vi "子VI-深度学习自动检测结果分析.vi"(2 "临界Z值":i32, 4 "临界面积百分比值":dbl, 6 "预测图片保存路径":path, 12 "产品规格":cluster{"产品长度（周长）（mm）":dbl, "产品宽度（母线长）（mm）":dbl}) -> (14 "弥散类检测结果":string[][](table), 17 "Threshold Image":T2(plugin-control), 18 "misan":T2(plugin-control), 19 "分层类检测结果":string[][](table))   [LabVIEW 2018]
uses:
  <vilib>/vision/NI_Vision_Development_Module.lvlib
panel:
  in  "Tab Control":T1
  out "?":T2(plugin-control)
  in  "格式字符串 3":string="%f"
  in  "分隔符（'\\'代码显示） 2":string="\t"
  out "弥散和分层临界灰度值":i64
  out "弥散缺陷个数":i32
  out "分层缺陷个数":i32
  out "合格？ 弥散类":string="fencengThreshold"
  out "合格？分层类":string="fencengThreshold"
  out "弥散测量结果":dbl[][](array[numeric]) format="%.2f"
  out "面积 (pixels)":i32
  in  "格式字符串 2":string="%f"
  in  "分隔符（'\\'代码显示）":string="\t"
  out "分层测量结果":dbl[][](array[numeric]) format="%.2f"
  out "缺陷初步分类的临界值":sgl format="%#.3f"
  # "所选区域信息"
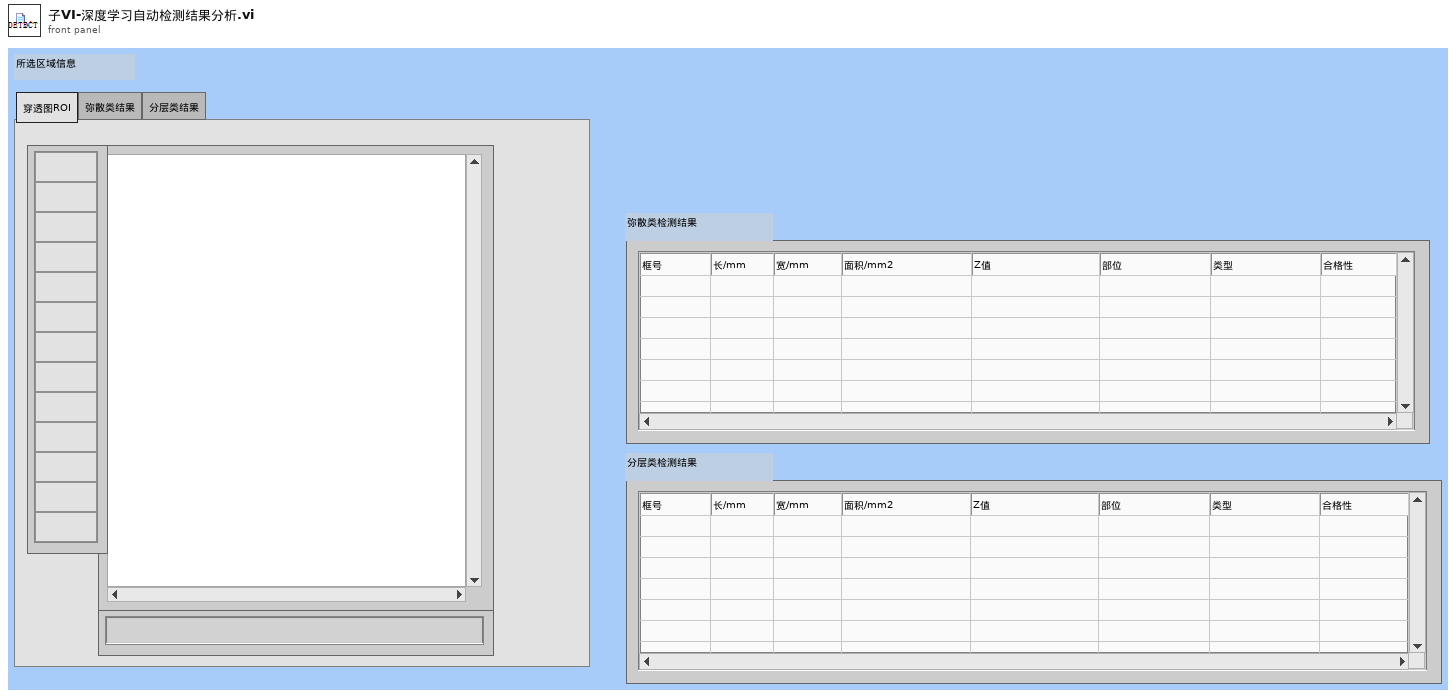
[diagram p1: front panel]
types:
  T1 = typedef "控件2.ctl" = enum32{"穿透图ROI", "弥散类结果", "分层类结果"}
  T2 = typedef "IMAQ Image.ctl" = refnum<image>
  T3 = typedef "Image Type" = u32
  T4 = typedef "Particle Parameters" = i32
  T5 = cluster{"Measurement Parameter":T4, "Range Lower Value":dbl, "Range Upper Value":dbl, "Range":bool, "Measurement Type":bool}[]
  T6 = cluster{"histogram":u32[], "Minimal Value":sgl, "Maximal Value":sgl, "Starting Value":sgl, "Interval Width":sgl, "Mean Value":sgl, "Standard  Variation":sgl, "Area (pixels)":i32}
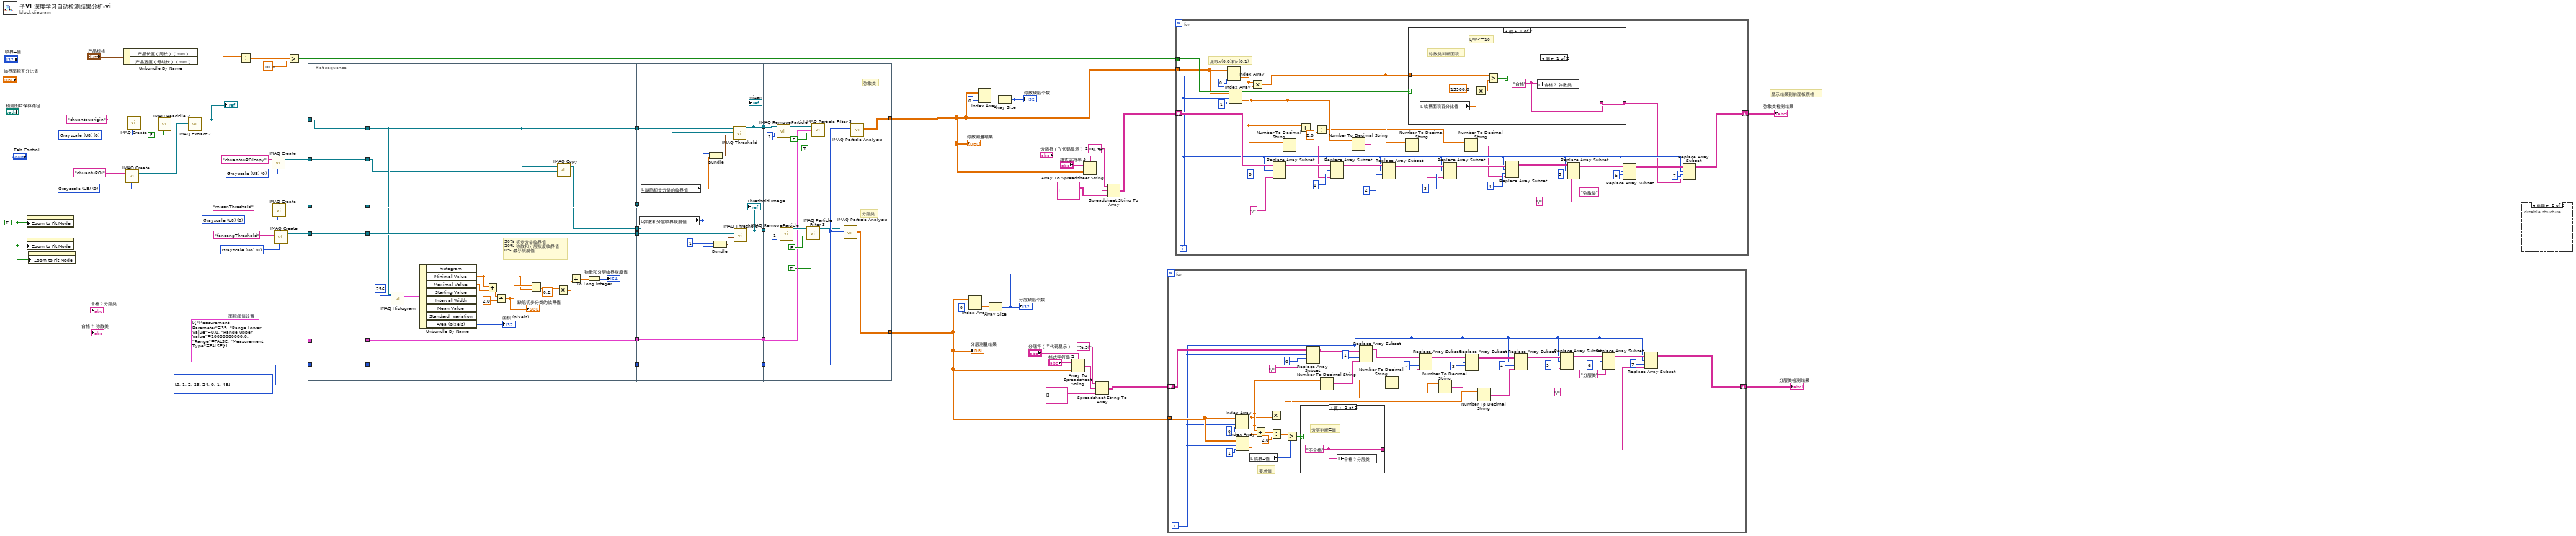
[diagram p0: block diagram]
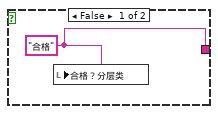
[diagram p2: hidden frame]
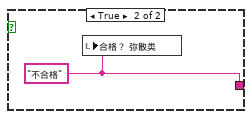
[diagram p3: hidden frame]
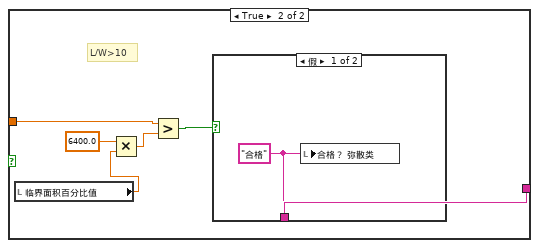
[diagram p4: hidden frame]
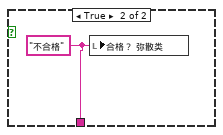
[diagram p5: hidden frame]
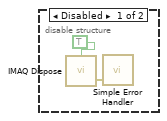
[diagram p6: hidden frame]
diagram:
  w1 = T3 0 items=["Grayscale (U8)", "Grayscale (I16)", "Grayscale (SGL)", "Complex (CSG)", "RGB (U32)", "HSL (U32)", "RGB (U64)", "Grayscale (U16)"] ("Image Type")
  w6 = TRUE ("Zoom to Fit Mode")
  w47 = T3 0 items=["Grayscale (U8)", "Grayscale (I16)", "Grayscale (SGL)", "Complex (CSG)", "RGB (U32)", "HSL (U32)", "RGB (U64)", "Grayscale (U16)"] ("Image Type")
  w48 = T3 0 items=["Grayscale (U8)", "Grayscale (I16)", "Grayscale (SGL)", "Complex (CSG)", "RGB (U32)", "HSL (U32)", "RGB (U64)", "Grayscale (U16)"] ("Image Type")
  w51 = T3 0 items=["Grayscale (U8)", "Grayscale (I16)", "Grayscale (SGL)", "Complex (CSG)", "RGB (U32)", "HSL (U32)", "RGB (U64)", "Grayscale (U16)"] ("Image Type")
  w29 = i32[] [0, 1, 2, 23, 24, 0, 1, 48] items=["Bounding Rect Width", "Bounding Rect Height"] ("Pixel Measurements")
  w33 = T5 [{"Measurement Parameter"=35, "Range Lower Value"=0.0, "Range Upper Value"=10000000000.0, "Range"=FALSE, "Measurement Type"=FALSE}]  # 面积阈值设置
  w65 = T3 0 items=["Grayscale (U8)", "Grayscale (I16)", "Grayscale (SGL)", "Complex (CSG)", "RGB (U32)", "HSL (U32)", "RGB (U64)", "Grayscale (U16)"] ("Image Type")
  # "显示结果到前面板表格"
  n1 = property class="ImageControl"("Zoom to Fit Mode"=w6) -> ()  [unwired: 2 in, 2 out]
  n2 = property class="ImageControl"("Zoom to Fit Mode"=w6) -> ()  [unwired: 2 in, 2 out]
  n3 = property class="ImageControl"("Zoom to Fit Mode"=w6) -> ()  [unwired: 2 in, 2 out]
  n4 = Unbundle By Name("产品规格") -> ("产品长度（周长）（mm）"=w59:dbl, "产品宽度（母线长）（mm）"=w58:dbl)
  n5 = call "IMAQ Create"("Image Name"="chuantuROI", "Image Type"=w51) -> ("New Image"=w50:T2)  [unwired: 3 in, 1 out]
  n6 = call "IMAQ Create"("Image Name"="chuantouorigin", "Image Type"=w65) -> ("New Image"=w53:T2)  [unwired: 3 in, 1 out]
  n7 = call "IMAQ ReadFile 2"("Use File Path Image Type"=FALSE, "File Path"="预测图片保存路径", "Image"=w53) -> ("Image Out"=w54:T2)  [unwired: 4 in, 4 out]
  n8 = call "IMAQ Extract 2"("Image Dst"=w50, "Image Src"=w54) -> ("Image Dst Out"=w9:T2)  [unwired: 8 in, 1 out]
  "?" <- w9
  n9 = Divide(x=w59, y=w58) -> (x/y=w62:dbl)
  n10 = call "IMAQ Create"("Image Name"="chuantouROIcopy", "Image Type"=w1) -> ("New Image"=w4:T2)  [unwired: 3 in, 1 out]
  n11 = call "IMAQ Create"("Image Name"="misanThreshold", "Image Type"=w47) -> ("New Image"=w40:T2)  [unwired: 3 in, 1 out]
  n12 = call "IMAQ Create"("Image Name"="fencengThreshold", "Image Type"=w48) -> ("New Image"=w38:T2)  [unwired: 3 in, 1 out]
  n13 = Greater?(x=w62, y=10.0) -> (0:w57:bool)
  n14 = flat-sequence {
    tunnel: w9 -> [w68]
    tunnel: w40 -> [w72]
    tunnel: [w72] -> w41
    tunnel: [w71] -> w39
    tunnel: w38 -> [w71]
    tunnel: [w70] -> w34
    tunnel: w33 -> [w70]
    tunnel: [w69] -> w30
    tunnel: w29 -> [w69]
    tunnel: [w68] -> w7
    tunnel: w4 -> [w67]
    tunnel: [w67] -> w3
    tunnel: [w92] -> w42
    tunnel: [w91] -> w37
    tunnel: [w86] -> w32
    tunnel: [w85] -> w28
    tunnel: w30 -> [w85]
    tunnel: w34 -> [w86]
    tunnel: w39 -> [w91]
    tunnel: w41 -> [w92]
    tunnel: [w75] -> w8
    tunnel: w7 -> [w75]
    tunnel: [w74] -> w5
    tunnel: w3 -> [w73]
    tunnel: w42 -> [w105]
    tunnel: w37 -> [w104]
    tunnel: [w94] -> w36
    tunnel: [w95] -> w35
    tunnel: w32 -> [w103]
    tunnel: [w103] -> w31
    tunnel: w28 -> [w102]
    tunnel: [w102] -> w27
    tunnel: w8 -> [w96]
    tunnel: w5 -> [w93]
    tunnel: [w108] -> w12
    tunnel: [w115] -> w20
    tunnel: w36 -> [w114]
    tunnel: w35 -> [w113]
    tunnel: w31 -> [w112]
    tunnel: w27 -> [w111]
    frame #0 {
    }
    frame #1 {
      # "50% 初步分类临界值\n20% 弥散和分层灰度临界值\n0% 最小灰度值"
      n15 = call "IMAQ Histogram"("Number of Classes"=256, "Image"=w75) -> ("Histogram Report"=w89:T6)  [unwired: 8 in, 1 out]
      n16 = Unbundle By Name(w89) -> ("Minimal Value"=w77:sgl, "Maximal Value"=w83:sgl, "Area (pixels)"=→"面积 (pixels)":i32)  [unwired: 5 out]
      n17 = Add(x=w77, y=w83) -> (x+y=w82:sgl)
      n18 = Divide(x=w82, y=sgl 2.0) -> (x/y=w81:sgl)
      "缺陷初步分类的临界值" <- w81
      n19 = Subtract(x=w81, y=w77) -> (x-y=w79:sgl)
      n20 = Multiply(x=w79, y=0.2) -> (x*y=w78:dbl)
      n21 = call "IMAQ Copy"("Image Dst"=w73, "Image Src"=w75) -> ("Image Dst Out"=w74:T2)  [unwired: 4 in, 1 out]
      n22 = Add(x=w77, y=w78) -> (x+y=w76:dbl)
      n23 = To Long Integer(number=w76) -> (32bit integer=→"弥散和分层临界灰度值":i32)
    }
    frame #2 {
      n24 = local read "弥散和分层临界灰度值"() -> (w98:i64)
      n25 = local read "缺陷初步分类的临界值"() -> (w100:sgl)
      n26 = Bundle("弥散和分层临界灰度值"=w98, "缺陷初步分类的临界值"=w100) -> (w101:cluster{"弥散和分层临界灰度值":i64, "缺陷初步分类的临界值":sgl})  [unwired: 1 in]
      n27 = Bundle(1, "弥散和分层临界灰度值"=w98) -> (w97:cluster{i32, "弥散和分层临界灰度值":i64})  [unwired: 1 in]
      n28 = call "IMAQ Threshold"("Range"=w101, "Image Dst"=w105, "Image Src"=w96) -> ("Image Dst Out"=w95:T2)  [unwired: 3 in, 5 out]
      "misan" <- w95
      n29 = call "IMAQ Threshold"("Range"=w97, "Image Dst"=w104, "Image Src"=w93) -> ("Image Dst Out"=w94:T2)  [unwired: 3 in, 5 out]
      "Threshold Image" <- w94
    }
    frame #3 {
      # "分层类"
      # "弥散类"
      n30 = call "IMAQ RemoveParticle"("Number of Erosion"=1, "Image Src"=w113) -> ("Image Dst Out"=w121:T2)  [unwired: 8 in, 1 out]
      n31 = call "IMAQ RemoveParticle"("Number of Erosion"=1, "Image Src"=w114) -> ("Image Dst Out"=w118:T2)  [unwired: 8 in, 1 out]
      n32 = call "IMAQ Particle Filter 3"("Image Src"=w118, "Keep/Remove Particles (F)"=FALSE, "Reject Border? (F)"=TRUE) -> ("Image Dst Out"=w109:T2)  [unwired: 10 in, 2 out]
      n33 = call "IMAQ Particle Filter 3"("Image Src"=w121, "Selection Values"=w112, "Keep/Remove Particles (F)"=FALSE, "Reject Border? (F)"=TRUE) -> ("Image Dst Out"=w110:T2)  [unwired: 9 in, 2 out]
      n34 = call "IMAQ Particle Analysis"("Pixel Measurements"=w111, "Image"=w109) -> ("Particle Measurements (Pixels)"=w115:dbl[][])  [unwired: 4 in, 5 out]
      n35 = call "IMAQ Particle Analysis"("Pixel Measurements"=w111, "Image"=w110) -> ("Particle Measurements (Pixels)"=w108:dbl[][])  [unwired: 4 in, 5 out]
    }
  }
  n36 = Index Array(array=w20, index (col)=0 ("禁用的索引 (列)")) -> (element=w46:dbl[])  [unwired: 1 in]
  n37 = Index Array(array=w12, index (col)=0 ("禁用的索引 (列)")) -> (element=w44:dbl[])  [unwired: 1 in]
  n38 = Array Size(array=w46) -> (size(s)=w26:i32)
  "分层缺陷个数" <- w26
  n39 = Array Size(array=w44) -> (size(s)=w56:i32)
  "弥散缺陷个数" <- w56
  n40 = Array To Spreadsheet String(delimiter (Tab)="分隔符（'\\'代码显示）", array=w20, 3:"格式字符串 2") -> (spreadsheet string=w23:string)
  n41 = Array To Spreadsheet String(delimiter (Tab)="分隔符（'\\'代码显示） 2", array=w12, 3:"格式字符串 3") -> (spreadsheet string=w15:string)
  n42 = Spreadsheet String To Array(format string="%.3f", spreadsheet string=w23, array type (2D Dbl)=string[][] [] ("Array")) -> (array=w19:string[][])  [unwired: 1 in]
  n43 = Spreadsheet String To Array(format string="%.3f", spreadsheet string=w15, array type (2D Dbl)=string[][] [] ("Array")) -> (array=w11:string[][])  [unwired: 1 in]
  n44 = for {
    N: w26 -> [_]
    tunnel: w20 -> [w152]
    shift-right: [w132] -> w18
    shift-left: w19 -> [w143]
    i -> [w127]
    # "要求值"
    n45 = Index Array(array=w152, index (row)=w127, index (col)=0 ("禁用的索引 (列)")) -> (element=w131:dbl)
    n46 = Index Array(array=w152, index (row)=w127, index (col)=1 ("禁用的索引 (列)")) -> (element=w130:dbl)
    n47 = local read "临界Z值"() -> (w156:i32)
    n48 = Add(x=w131, y=w130) -> (x+y=w157:dbl)
    n49 = Multiply(x=w131, y=w130) -> (x*y=w129:dbl)
    n50 = Divide(x=w157, y=2.0) -> (x/y=w126:dbl)
    n51 = Greater?(x=w126, y=w156) -> (0:w158:bool)
    n52 = case shown="真" w158 {
      tunnel: [w159 w160] -> w124
      frame False {
        w159 = "合格" ("合格？")
        n53 = local write "合格？分层类"(w159) -> ()
      }
      frame True {
        w160 = "不合格" ("合格？")
        # "分层判断Z值"
        n54 = local write "合格？分层类"(w160) -> ()
      }
    }
    n55 = Replace Array Subset(array=w143, new element="/" ("新元素/子数组"), index (row)=w127, index (col)=0 ("索引 (列)")) -> (w142:string[][])
    n56 = Number To Decimal String(number=w131) -> (decimal integer string=w141:string)  [unwired: 1 in]
    n57 = Replace Array Subset(array=w142, new element=w141, index (row)=w127, index (col)=1 ("索引 (列)")) -> (w139:string[][])
    n58 = Number To Decimal String(number=w130) -> (decimal integer string=w140:string)  [unwired: 1 in]
    n59 = Replace Array Subset(array=w139, new element=w140, index (row)=w127, index (col)=2 ("索引 (列)")) -> (w138:string[][])
    n60 = Number To Decimal String(number=w129) -> (decimal integer string=w137:string)  [unwired: 1 in]
    n61 = Replace Array Subset(array=w138, new element=w137, index (row)=w127, index (col)=3 ("索引 (列)")) -> (w136:string[][])
    n62 = Number To Decimal String(number=w126) -> (decimal integer string=w128:string)  [unwired: 1 in]
    n63 = Replace Array Subset(array=w136, new element=w128, index (row)=w127, index (col)=4 ("索引 (列)")) -> (w135:string[][])
    n64 = Replace Array Subset(array=w135, new element="/" ("新元素/子数组"), index (row)=w127, index (col)=5 ("索引 (列)")) -> (w134:string[][])
    n65 = Replace Array Subset(array=w134, new element="分层类" ("新元素/子数组"), index (row)=w127, index (col)=6 ("索引 (列)")) -> (w133:string[][])
    n66 = Replace Array Subset(array=w133, new element=w124, index (row)=w127, index (col)=7 ("索引 (列)")) -> (w132:string[][])
  }
  "分层类检测结果" <- w18
  n67 = for {
    N: w56 -> [_]
    tunnel: w57 -> [w196]
    tunnel: w12 -> [w195]
    shift-right: [w176] -> w10
    shift-left: w11 -> [w184]
    i -> [w174]
    # "提取x(0,0)和y(0,1)"
    n68 = Index Array(array=w195, index (row)=w174, index (col)=0 ("禁用的索引 (列)")) -> (element=w168:dbl)
    n69 = Index Array(array=w195, index (row)=w174, index (col)=1 ("禁用的索引 (列)")) -> (element=w167:dbl)
    n70 = Multiply(x=w168, y=w167) -> (x*y=w172:dbl)
    n71 = Replace Array Subset(array=w184, new element="/" ("新元素/子数组"), index (row)=w174, index (col)=0 ("索引 (列)")) -> (w183:string[][])
    n72 = Number To Decimal String(number=w168) -> (decimal integer string=w175:string)  [unwired: 1 in]
    n73 = Add(x=w168, y=w167) -> (x+y=w170:dbl)
    n74 = Divide(x=w170, y=2.0) -> (x/y=w166:dbl)
    n75 = Replace Array Subset(array=w183, new element=w175, index (row)=w174, index (col)=1 ("索引 (列)")) -> (w182:string[][])
    n76 = Number To Decimal String(number=w167) -> (decimal integer string=w173:string)  [unwired: 1 in]
    n77 = Replace Array Subset(array=w182, new element=w173, index (row)=w174, index (col)=2 ("索引 (列)")) -> (w181:string[][])
    n78 = Number To Decimal String(number=w172) -> (decimal integer string=w171:string)  [unwired: 1 in]
    n79 = case shown="假" w196 {
      tunnel: w172 -> [w202 w210]
      tunnel: [w200 w208] -> w163
      frame False {
        # "弥散类判断面积"
        # "L/W<=10"
        n80 = local read "临界面积百分比值"() -> (w198:dbl)
        n81 = Multiply(x=15500.0, y=w198) -> (x*y=w197:dbl)
        n82 = Greater?(x=w202, y=w197) -> (0:w201:bool)
        n83 = case shown="假" w201 {
          tunnel: [w203 w204] -> w200
          frame False {
            w203 = "合格" ("合格？")
            n84 = local write "合格？ 弥散类"(w203) -> ()
          }
          frame True {
            w204 = "不合格" ("合格？")
            n85 = local write "合格？ 弥散类"(w204) -> ()
          }
        }
      }
      frame True {
        # "L/W>10"
        n86 = local read "临界面积百分比值"() -> (w205:dbl)
        n87 = Multiply(x=6400.0, y=w205) -> (x*y=w207:dbl)
        n88 = Greater?(x=w210, y=w207) -> (0:w209:bool)
        n89 = case shown="假" w209 {
          tunnel: [w211 w212] -> w208
          frame False {
            w211 = "合格" ("合格？")
            n90 = local write "合格？ 弥散类"(w211) -> ()
          }
          frame True {
            w212 = "不合格" ("合格？")
            n91 = local write "合格？ 弥散类"(w212) -> ()
          }
        }
      }
    }
    n92 = Replace Array Subset(array=w181, new element=w171, index (row)=w174, index (col)=3 ("索引 (列)")) -> (w180:string[][])
    n93 = Number To Decimal String(number=w166) -> (decimal integer string=w165:string)  [unwired: 1 in]
    n94 = Replace Array Subset(array=w180, new element=w165, index (row)=w174, index (col)=4 ("索引 (列)")) -> (w179:string[][])
    n95 = Replace Array Subset(array=w179, new element="/" ("新元素/子数组"), index (row)=w174, index (col)=5 ("索引 (列)")) -> (w178:string[][])
    n96 = Replace Array Subset(array=w178, new element="弥散类" ("新元素/子数组"), index (row)=w174, index (col)=6 ("索引 (列)")) -> (w177:string[][])
    n97 = Replace Array Subset(array=w177, new element=w163, index (row)=w174, index (col)=7 ("索引 (列)")) -> (w176:string[][])
  }
  "弥散类检测结果" <- w10
  n98 = disable-structure shown="启用" {
    frame Disabled {
      n99 = call "IMAQ Dispose"("All Images? (No)"=TRUE) -> ("error out"=w214:errorcluster)  [unwired: 5 in]
      n100 = call <vilib>:"Simple Error Handler.vi"("error in (no error)"=w214) -> ()  [unwired: 4 in, 5 out]
    }
    frame Enabled {
    }
  }
  "分层测量结果" <- w20
  "弥散测量结果" <- w12
